vi "NM GlobalTest.vi"() -> ()   [LabVIEW 2010] (continued)
          n20 = Select(t=4, s="Timing", f=0) -> (s? t:f=w5836:i32)
        }
        frame 5 {
          # "TRIGGERING"
          n21 = Select(t=5, s="Trig", f=0) -> (s? t:f=w5841:i32)
        }
        frame 6 {
          # "START"
          n22 = Select(t=6, s="Start", f=0) -> (s? t:f=w5846:i32)
        }
        frame 7 {
          # "WRITE"
          n23 = Select(t=7, s="Write", f=0) -> (s? t:f=w5851:i32)
        }
        frame 8 {
          # "IDLE and UPDATE CONTROLS"
          n24 = Select(t=1, s="Idle 2", f=0) -> (s? t:f=w5856:i32)
        }
        frame 9 {
          # "READ"
          n25 = Select(t=11, s="Read", f=0) -> (s? t:f=w5861:i32)
        }
        frame 10 {
          # "START"
          n26 = Select(t=6, s="Start", f=0) -> (s? t:f=w5867:i32)
        }
        frame 11 {
          # "STATUS"
          n27 = Select(t=8, s="Status\nLoop", f=0) -> (s? t:f=w5873:i32)
        }
        frame 12 {
          # "Property Nodes"
          n28 = Select(t=13, s="Props", f=0) -> (s? t:f=w5877:i32)
        }
        frame 13 {
          # "WAIT"
          n29 = Select(t=12, s="Wait", f=0) -> (s? t:f=w5882:i32)
        }
        frame 14 {
          # "STOP"
          n30 = Select(t=9, s="Stop", f=0) -> (s? t:f=w5888:i32)
        }
        frame 15 {
          # "CLEAR"
          n31 = case shown="\"ULx\", Default" w5893 {
            tunnel: w5894 -> [w5900 _]
            tunnel: w5895 -> [_ w5903]
            frame "ULx", Default {
              n32 = call "ULxTaskInfo.vi"("task in"=w5900) -> ("Task"=w5901:i32)  [unwired: 2 out]
              n33 = local write "Task"(w5901) -> ()
            }
            frame "DAQmx" {
              n34 = call "DAQmxTaskInfo.vi"("task in"=w5903) -> ("Name"=w5902:refnum<k21>)  [unwired: 1 out]
              n35 = local write "Name"(w5902) -> ()
            }
          }
          n36 = call "TextError.vi"("error in"=w5891) -> ("message"=w5892:string)  [unwired: 1 in]
          n37 = local write "message 2"(w5892) -> ()
          n38 = Select(t=10, s="Clear", f=0) -> (s? t:f=w5897:i32)
        }
        frame 16 {
          # "Task Control"
          n39 = Select(t=14, s="NI\nTC", f=0) -> (s? t:f=w5904:i32)
        }
        frame 17 {
          n40 = case shown="True" "Clear\nError" {
            tunnel: w5910 -> [w5913 w5915]
            tunnel: [w5913 w5914] -> w5909
            frame False {
            }
            frame True {
              n41 = local write "Clear\nError"(FALSE) -> ()
              n42 = call <vilib>:"Clear Errors.vi"("error in (no error)"=w5915) -> ("error out"=w5914:errorcluster)  [unwired: 6 in]
            }
          }
        }
      }
      n43 = case shown="13" w33 {
        tunnel: "SelLib" -> [_ _ w155 w1018 w1069 w1147 w1386 w1435 w2708 w2768 w2791 w2812 w3897 w3943 w5784]
        tunnel: w22 -> [w47 w54 w153 w1024 w1068 w1148 w1395 w1434 w2714 w2767 w2794 w2815 w3901 w3940 w5788]
        tunnel: w23 -> [w46 w53 w154 w1023 w1067 w1150 w1394 w1433 w2713 w2766 w2793 w2814 w3902 w3941 w5786]
        tunnel: [w47 w52 w150 w1021 w1065 w1158 w1385 w1431 w2711 w2764 w2789 w2811 w3900 w3938 w5787] -> w35
        tunnel: [w46 w51 w151 w1020 w1064 w1157 w1384 w1430 w2710 w2763 w2788 w2810 w3899 w3937 w5783] -> w34
        tunnel: [w45 _ w152 w1019 w1063 w1156 w1383 w1429 w2709 w2762 w2787 w2809 w3898 w3939 w5782] -> w32
        tunnel: w16 -> [w45 _ _ w1022 w1066 w1149 w1393 w1432 w2712 w2765 w2792 w2813 w3903 w3942 w5785]
        tunnel: "Item" -> [_ _ w146 _ w1061 w1145 w1391 w1428 w2707 w2760 w2785 w2808 w3892 w3936 w5779]
        tunnel: w19 -> [_ w50 _ _ _ _ w1390 _ _ _ _ _ _ _ _]
        tunnel: w17 -> [w40 _ _ _ _ _ _ _ _ _ _ _ _ _ _]
        frame ..0, Default {
          # "Do Nothing"
          n44 = First Call?() -> (First Call?: T/F=w38:bool)
          n45 = Or(x=w38, y=w40) -> (x .or. y?=w39:bool)
          n46 = case shown="False" w39 {
            frame False {
            }
            frame True {
              n47 = local read "SelLib"() -> (w48:enum32{"ULx", "DAQmx"})
              n48 = local write "AChan"(w48) -> ()
              n49 = local write "TrgEdge"(w48) -> ()
              n50 = local write "DChan"(w48) -> ()
              n51 = local write "CtrChan"(w48) -> ()
              n52 = local write "CompIn"(w48) -> ()
              n53 = local write "CompOut"(w48) -> ()
              n54 = local write "TmgImp"(w48) -> ()
              n55 = local write "TmgWfm"(w48) -> ()
              n56 = local write "UDClock"(w48) -> ()
              n57 = local write "SetWProps"(w48) -> ()
              n58 = local write "GetWProps"(w48) -> ()
              n59 = local write "GetCOPrp"(w48) -> ()
              n60 = local write "TrigLib"(w48) -> ()
              n61 = local write "GetCiPrp"(w48) -> ()
              n62 = local write "GetTmgPrp"(w48) -> ()
            }
          }
          n63 = local read "Timing"() -> (w43:bool)
          n64 = local read "Write"() -> (w44:bool)
          n65 = local read "Props"() -> (w37:bool)
          n66 = local read "Trig"() -> (w42:bool)
          n67 = local read "Read"() -> (w41:bool)
          n68 = property on="GetSet" class="TabCtl (strict)"("Visible"=w37) -> ()  [unwired: 2 in, 2 out]
          n69 = property on="TrigType" class="TabCtl (strict)"("Visible"=w42) -> ()  [unwired: 2 in, 2 out]
          n70 = property on="Tab Control" class="TabCtl (strict)"("Visible"=w43) -> ()  [unwired: 2 in, 2 out]
          n71 = property on="TaskType 2" class="TabCtl (strict)"("Visible"=w44) -> ()  [unwired: 2 in, 2 out]
          n72 = property on="ReadType" class="TabCtl (strict)"("Visible"=w41) -> ()  [unwired: 2 in, 2 out]
        }
        frame 1 {
          # "IDLE and UPDATE CONTROLS"
          n73 = while {
            shift-right: [w80] -> _
            shift-left: _ -> [w97]
            tunnel: [FALSE ("f")] -> w49
            tunnel: w54 -> [w85]
            tunnel: w53 -> [w84]
            tunnel: [w79] -> w52
            tunnel: [w68] -> w51
            tunnel: w50 -> [w73]
            stop <- w100 stop-if-true
            n74 = case shown="0, Default" w73 {
              tunnel: ["Clear" "Clear"] -> w91
              tunnel: ["Stop" "Stop"] -> w90
              tunnel: ["Start" "Start"] -> w89
              frame 0, Default {
              }
              frame 1 {
              }
            }
            n75 = local read "SelLib"() -> (w69:enum32{"ULx", "DAQmx"})
            n76 = Not(x="Plots") -> (.not. x?=w58:bool)
            n77 = local write "UDClock"(w69) -> ()
            n78 = local write "TmgWfm"(w69) -> ()
            n79 = local write "TmgImp"(w69) -> ()
            n80 = property on="DblPlot" class="WFGraph (strict)"("Visible"="Plots") -> ()  [unwired: 2 in, 2 out]
            n81 = property on="u32Plot" class="WFGraph (strict)"("Visible"="Plots") -> ()  [unwired: 2 in, 2 out]
            n82 = property on="u32Array" class="Arr (strict)"("Visible"=w58) -> ()  [unwired: 2 in, 2 out]
            n83 = property on="DblArray 2" class="Arr (strict)"("Visible"=w58) -> ()  [unwired: 2 in, 2 out]
            n84 = call "NMIdleLoop.vi"("mx task in"=w85, "ULx task in"=w84, "Tab Control"=w69, "Start"=w89, "ExStop"=w90, "ExClear"=w91) -> ("Task Start"=w86:bool, "Task Stop"=w87:bool, "Task Clear"=w88:bool, "mx task out"=w79:refnum<k21>, "ULx task out"=w68:refnum<k24>, "Name"=w81:refnum<k21>, "Task"=w77:i32, "Function"=w82:i32, "error out"=w56:errorcluster)  [unwired: 5 in]
            n85 = Compound Arithmetic op=OR(w88, w87, w86) -> (w83:bool)
            n86 = local write "TrgEdge"(w69) -> ()
            n87 = local write "AChan"(w69) -> ()
            n88 = local write "CompOut"(w69) -> ()
            n89 = local write "Name"(w81) -> ()
            n90 = local read "Write"() -> (w92:bool)
            n91 = local read "Read"() -> (w74:bool)
            n92 = local read "Timing"() -> (w76:bool)
            n93 = local read "Trig"() -> (w75:bool)
            n94 = local write "CtrChan"(w69) -> ()
            n95 = local write "DChan"(w69) -> ()
            n96 = local write "CompIn"(w69) -> ()
            n97 = property on="ReadType" class="TabCtl (strict)"("Visible"=w74) -> ()  [unwired: 2 in, 2 out]
            n98 = property on="TaskType 2" class="TabCtl (strict)"("Visible"=w92) -> ()  [unwired: 2 in, 2 out]
            n99 = property on="Tab Control" class="TabCtl (strict)"("Visible"=w76) -> ()  [unwired: 2 in, 2 out]
            n100 = property on="TrigType" class="TabCtl (strict)"("Visible"=w75) -> ()  [unwired: 2 in, 2 out]
            n101 = local write "Task"(w77) -> ()
            n102 = case shown="\"DAQmx\"" w69 {
              tunnel: w79 -> [_ w125]
              tunnel: w77 -> [w117 _]
              tunnel: w68 -> [w116 _]
              tunnel: [w112 w120] -> w57
              tunnel: w56 -> [w111 w123]
              tunnel: [w110 w124] -> w55
              frame "ULx", Default {
                n103 = Equal To 0?(x=w117) -> (x = 0?=w118:bool)
                n104 = call <vilib>:"ULx Is Task Done.vi"("task in"=w116, "error in"=w111) -> ("task done?"=w115:bool, "error out"=w110:errorcluster)  [unwired: 11 in, 1 out]
                n105 = local write "Task Cleared"(w118) -> ()
                n106 = local write "Task Stopped"(w115) -> ()
                n107 = Unbundle By Name(w110) -> ("code"=w114:i32)
                n108 = Not Equal?(x=w114, y=100000) -> (x != y?=w112:bool)
              }
              frame "DAQmx" {
                n109 = call <vilib>:"DAQmx Is Task Done.vi"("task/channels in"=w125, "error in"=w123) -> ("task done?"=w122:bool, "error out"=w124:errorcluster)  [unwired: 11 in, 1 out]
                n110 = Unbundle By Name(w124) -> ("code"=w127:i32)
                n111 = Equal?(x=w127, y=-200088) -> (x = y?=w119:bool)
                n112 = Or(x=w122, y=w119) -> (x .or. y?=w121:bool)
                n113 = Not(x=w119) -> (.not. x?=w120:bool)
                n114 = local write "Task Stopped"(w121) -> ()
                n115 = local write "Task Cleared"(w119) -> ()
              }
            }
            n116 = case shown="0, Default" w82 {
              tunnel: w69 -> [_ w129 w132 _]
              tunnel: w77 -> [_ _ _ _]
              frame 0, Default {
              }
              frame 1 {
                w128 = FALSE ("Start 2")
                n117 = case shown="\"ULx\", Default" w129 {
                  frame "ULx", Default {
                    n118 = local write "Task Stopped"(FALSE ("Task Stopped")) -> ()
                  }
                  frame "DAQmx" {
                  }
                }
                n119 = local write "Start"(w128) -> ()
                n120 = local write "Start"(w128) -> ()
              }
              frame 2 {
                w131 = FALSE ("Stop")
                n121 = case shown="\"ULx\", Default" w132 {
                  frame "ULx", Default {
                    n122 = local write "Task Stopped"(TRUE ("Task Stopped")) -> ()
                  }
                  frame "DAQmx" {
                  }
                }
                n123 = local write "Stop"(w131) -> ()
                n124 = local write "Stop"(w131) -> ()
              }
              frame 3 {
                w134 = FALSE ("Clear")
                n125 = local write "Clear"(w134) -> ()
                n126 = local write "Clear"(w134) -> ()
              }
            }
            n127 = local write "GetWProps"(w69) -> ()
            n128 = local write "SetWProps"(w69) -> ()
            n129 = local write "TrigLib"(w69) -> ()
            n130 = local read "Mod Array"() -> (w64:bool)
            n131 = local write "GetTmgPrp"(w69) -> ()
            n132 = local write "GetCOPrp"(w69) -> ()
            n133 = property on="digital data 3" class="Arr (strict)"("Visible"="Dig/Ctr") -> ()  [unwired: 2 in, 2 out]
            n134 = local write "GetCiPrp"(w69) -> ()
            n135 = property on="DataGen" class="TabCtl (strict)"("Visible"="Data") -> ()  [unwired: 2 in, 2 out]
            n136 = property on="Tab Control 3" class="TabCtl (strict)"("Visible"=w64) -> ()  [unwired: 2 in, 2 out]
            n137 = Not(x="Dig/Ctr") -> (.not. x?=w61:bool)
            n138 = local read "Idle 2"() -> (w71:bool)
            n139 = local read "Idle"() -> (w78:bool)
            n140 = local read "Props"() -> (w70:bool)
            n141 = Not(x=w97) -> (.not. x?=w95:bool)
            n142 = property on="counter data" class="Arr (strict)"("Visible"=w61) -> ()  [unwired: 2 in, 2 out]
            n143 = Wait Until Next ms Multiple(millisecond multiple=u32 200) -> ()  [unwired: 1 out]
            n144 = property on="GetSet" class="TabCtl (strict)"("Visible"=w70) -> ()  [unwired: 2 in, 2 out]
            n145 = Or(x=w71, y=w78) -> (x .or. y?=w72:bool)
            n146 = case shown="Error" w55 {
              selector: w55 -> [w135 w140]
              tunnel: w83 -> [w136 _]
              tunnel: w57 -> [_ w139]
              frame No Error {
                n147 = case shown="True" w136 {
                  tunnel: w135 -> [_ w138]
                  frame False {
                  }
                  frame True {
                    n148 = call "TextError.vi"("error in"=w138) -> ("message"=w137:string)  [unwired: 1 in]
                    n149 = local write "message 2"(w137) -> ()
                  }
                }
              }
              frame Error {
                n150 = case shown="True" w139 {
                  tunnel: w140 -> [_ w142]
                  frame False {
                  }
                  frame True {
                    n151 = call "TextError.vi"("error in"=w142) -> ("message"=w141:string)  [unwired: 1 in]
                    n152 = local write "message 2"(w141) -> ()
                  }
                }
              }
            }
            n153 = local read "stop"() -> (w96:bool)
            n154 = Not(x=w72) -> (.not. x?=w98:bool)
            n155 = Select(t=w95, s=w72, f=FALSE) -> (s? t:f=w80:bool)
            n156 = Not(x="Show Plot") -> (.not. x?=w62:bool)
            n157 = Not(x="Show Plot") -> (.not. x?=w65:bool)
            n158 = property on="DblArray" class="WFGraph (strict)"("Visible"="Show Plot") -> ()  [unwired: 2 in, 2 out]
            n159 = case shown="0, Default" w73 {
              tunnel: w80 -> [w108 w109]
              frame 0, Default {
                "Idle" <- w108
              }
              frame 1 {
                "Idle 3" <- w109
              }
            }
            n160 = property on="data 41" class="Arr (strict)"("Visible"=w65) -> ()  [unwired: 2 in, 2 out]
            n161 = Compound Arithmetic op=OR(w96, w98, "Submit") -> (w100:bool)
            n162 = property on="data 7" class="Arr (strict)"("Visible"=w62) -> ()  [unwired: 2 in, 2 out]
            n163 = property on="data 76" class="WFGraph (strict)"("Visible"="Show Plot") -> ()  [unwired: 2 in, 2 out]
          }
          n164 = local write "Idle"(w49) -> ()
          n165 = local write "Idle 3"(w49) -> ()
          n166 = local write "Submit"(w49) -> ()
        }
        frame 2 {
          # "CREATE CHANNELS"
          n167 = case shown="\"Counter\"" "TaskType" {
            tunnel: [w169 w401 w483 w835 w948] -> w151
            tunnel: [w168 w400 w485 w836 w950] -> w149
            tunnel: [w167 w399 w484 w837 w949] -> w148
            tunnel: w155 -> [w166 w398 w482 _ _]
            tunnel: [w165 w397 w481 w834 w947] -> w150
            tunnel: w153 -> [w164 w395 w480 w834 w947]
            tunnel: w154 -> [w163 w396 w479 _ _]
            tunnel: [w162 w394 w478 w833 w946] -> w143
            frame "Analog", Default {
              n168 = case shown="\"DAQmx\"" w166 {
                tunnel: [w176 w279] -> w169
                tunnel: [w175 w282] -> w168
                tunnel: [w174 w281] -> w167
                tunnel: [w173 w280] -> w165
                tunnel: w164 -> [w173 _]
                tunnel: w163 -> [_ w279]
                tunnel: [w172 ""] -> w162
                tunnel: [w171 w277] -> w157
                tunnel: [w170 w276] -> w156
                frame "ULx", Default {
                  n169 = case shown="\"AO Volts\"" "AnalogType" {
                    tunnel: [w183 w210 w228 w247 w266] -> w174
                    tunnel: [w182 w211 w229 w248 w267] -> w175
                    tunnel: [w181 w217 w235 w254 w273] -> w176
                    tunnel: ["ULx" "ULx" "ULx" "ULx" "ULx"] -> w172
                    tunnel: [-5.0 ("min") -5.0 ("min") -5.0 ("min") "min" "min"] -> w170
                    tunnel: [5.0 ("max") 5.0 ("max") 5.0 ("max") "max" "max"] -> w171
                    frame "AI Volts", Default {
                      n170 = call-poly <vilib>:"ULx Create Virtual Channel.vi"("maximum value"="max", "minimum value"="min", "physical channels"="ULx") -> ("task out"=w198:refnum<k24>, "error out"=w188:errorcluster)  [unwired: 11 in]
                      n171 = call "TrapBlankChan.vi"("error in (no error)"=w188) -> ("error out"=w187:errorcluster)  [unwired: 9 in, 1 out]
                      n172 = call-poly <vilib>:"ULx Create Virtual Channel.vi"("task in"=w198, "maximum value"="max 2", "minimum value"="min 2", "physical channels"="physical channels 2", "error in"=w187) -> ("task out"=w197:refnum<k24>, "error out"=w186:errorcluster)  [unwired: 9 in]
                      n173 = call "TrapBlankChan.vi"("error in (no error)"=w186) -> ("error out"=w185:errorcluster)  [unwired: 9 in, 1 out]
                      n174 = call-poly <vilib>:"ULx Create Virtual Channel.vi"("task in"=w197, "maximum value"="max 3", "minimum value"="min 3", "physical channels"="physical channels 3", "error in"=w185) -> ("task out"=w181:refnum<k24>, "error out"=w184:errorcluster)  [unwired: 9 in]
                      n175 = call "TrapBlankChan.vi"("error in (no error)"=w184) -> ("message"=w183:string, "error out"=w182:errorcluster)  [unwired: 9 in]
                    }
                    frame "AI Cur" {
                      n176 = call-poly <vilib>:"ULx Create Virtual Channel.vi"("maximum value"="max", "minimum value"="min", "physical channels"="ULx") -> ("task out"=w219:refnum<k24>, "error out"=w216:errorcluster)  [unwired: 11 in]
                      n177 = call "TrapBlankChan.vi"("error in (no error)"=w216) -> ("error out"=w215:errorcluster)  [unwired: 9 in, 1 out]
                      n178 = call-poly <vilib>:"ULx Create Virtual Channel.vi"("task in"=w219, "maximum value"="max 4", "minimum value"="min 4", "physical channels"="physical channels 5", "error in"=w215) -> ("task out"=w218:refnum<k24>, "error out"=w214:errorcluster)  [unwired: 9 in]
                      n179 = call "TrapBlankChan.vi"("error in (no error)"=w214) -> ("error out"=w213:errorcluster)  [unwired: 9 in, 1 out]
                      n180 = call-poly <vilib>:"ULx Create Virtual Channel.vi"("task in"=w218, "maximum value"="max 5", "minimum value"="min 5", "physical channels"="physical channels 6", "error in"=w213) -> ("task out"=w217:refnum<k24>, "error out"=w212:errorcluster)  [unwired: 9 in]
                      n181 = call "TrapBlankChan.vi"("error in (no error)"=w212) -> ("message"=w210:string, "error out"=w211:errorcluster)  [unwired: 9 in]
                    }
                    frame "AI Temp" {
                      n182 = call-poly <vilib>:"ULx Create Virtual Channel.vi"("physical channels"="ULx", "units"="units") -> ("task out"=w237:refnum<k24>, "error out"=w234:errorcluster)  [unwired: 12 in]
                      n183 = call "TrapBlankChan.vi"("error in (no error)"=w234) -> ("error out"=w233:errorcluster)  [unwired: 9 in, 1 out]
                      n184 = call-poly <vilib>:"ULx Create Virtual Channel.vi"("task in"=w237, "physical channels"="physical channels 8", "units"="units 2", "error in"=w233) -> ("task out"=w236:refnum<k24>, "error out"=w232:errorcluster)  [unwired: 10 in]
                      n185 = call "TrapBlankChan.vi"("error in (no error)"=w232) -> ("error out"=w231:errorcluster)  [unwired: 9 in, 1 out]
                      n186 = call-poly <vilib>:"ULx Create Virtual Channel.vi"("task in"=w236, "physical channels"="physical channels 9", "units"="units 3", "error in"=w231) -> ("task out"=w235:refnum<k24>, "error out"=w230:errorcluster)  [unwired: 10 in]
                      n187 = call "TrapBlankChan.vi"("error in (no error)"=w230) -> ("message"=w228:string, "error out"=w229:errorcluster)  [unwired: 9 in]
                    }
                    frame "AO Volts" {
                      n188 = call-poly <vilib>:"ULx Create Virtual Channel.vi"("maximum value"="max", "minimum value"="min", "physical channels"="ULx") -> ("task out"=w256:refnum<k24>, "error out"=w253:errorcluster)  [unwired: 11 in]
                      n189 = call "TrapBlankChan.vi"("error in (no error)"=w253) -> ("error out"=w252:errorcluster)  [unwired: 9 in, 1 out]
                      n190 = call-poly <vilib>:"ULx Create Virtual Channel.vi"("task in"=w256, "maximum value"="max 8", "minimum value"="min 8", "physical channels"="physical channels 11", "error in"=w252) -> ("task out"=w255:refnum<k24>, "error out"=w251:errorcluster)  [unwired: 9 in]
                      n191 = call "TrapBlankChan.vi"("error in (no error)"=w251) -> ("error out"=w250:errorcluster)  [unwired: 9 in, 1 out]
                      n192 = call-poly <vilib>:"ULx Create Virtual Channel.vi"("task in"=w255, "maximum value"="max 7", "minimum value"="min 7", "physical channels"="physical channels 12", "error in"=w250) -> ("task out"=w254:refnum<k24>, "error out"=w249:errorcluster)  [unwired: 9 in]
                      n193 = call "TrapBlankChan.vi"("error in (no error)"=w249) -> ("message"=w247:string, "error out"=w248:errorcluster)  [unwired: 9 in]
                    }
                    frame "AO Cur" {
                      n194 = call-poly <vilib>:"ULx Create Virtual Channel.vi"("maximum value"="max", "minimum value"="min", "physical channels"="ULx") -> ("task out"=w275:refnum<k24>, "error out"=w272:errorcluster)  [unwired: 11 in]
                      n195 = call "TrapBlankChan.vi"("error in (no error)"=w272) -> ("error out"=w271:errorcluster)  [unwired: 9 in, 1 out]
                      n196 = call-poly <vilib>:"ULx Create Virtual Channel.vi"("task in"=w275, "maximum value"="max 11", "minimum value"="min 11", "physical channels"="physical channels 14", "error in"=w271) -> ("task out"=w274:refnum<k24>, "error out"=w270:errorcluster)  [unwired: 9 in]
                      n197 = call "TrapBlankChan.vi"("error in (no error)"=w270) -> ("error out"=w269:errorcluster)  [unwired: 9 in, 1 out]
                      n198 = call-poly <vilib>:"ULx Create Virtual Channel.vi"("task in"=w274, "maximum value"="max 10", "minimum value"="min 10", "physical channels"="physical channels 15", "error in"=w269) -> ("task out"=w273:refnum<k24>, "error out"=w268:errorcluster)  [unwired: 9 in]
                      n199 = call "TrapBlankChan.vi"("error in (no error)"=w268) -> ("message"=w266:string, "error out"=w267:errorcluster)  [unwired: 9 in]
                    }
                  }
                }
                frame "DAQmx" {
                  n200 = case shown="\"AI Volts\", Default" "xAnalog\nType" {
                    tunnel: [w289 w316 w344 w373 w392] -> w281
                    tunnel: [w290 w317 w350 w374 w393] -> w282
                    tunnel: [w292 w324 w349 w367 w388] -> w280
                    tunnel: [5.0 ("max") 5.0 ("max") 5.0 ("max") "max" "max"] -> w277
                    tunnel: [-5.0 ("min") -5.0 ("min") -5.0 ("min") "min" "min"] -> w276
                    frame "AI Volts", Default {
                      n201 = call-poly <vilib>:"DAQmx Create Virtual Channel.vi"("maximum value"="max", "minimum value"="min", "physical channels"="DAQmx", "name to assign"="name 1") -> ("task out"=w302:refnum<k21>, "error out"=w307:errorcluster)  [unwired: 10 in]
                      n202 = call "NITrapBlankChan.vi"("error in (no error)"=w307) -> ("error out"=w303:errorcluster)  [unwired: 9 in, 1 out]
                      n203 = call-poly <vilib>:"DAQmx Create Virtual Channel.vi"("task in"=w302, "maximum value"="max 19", "minimum value"="min 19", "physical channels"="physical channels 32", "name to assign"="name 2", "error in"=w303) -> ("task out"=w298:refnum<k21>, "error out"=w297:errorcluster)  [unwired: 8 in]
                      n204 = call "NITrapBlankChan.vi"("error in (no error)"=w297) -> ("error out"=w296:errorcluster)  [unwired: 9 in, 1 out]
                      n205 = call-poly <vilib>:"DAQmx Create Virtual Channel.vi"("task in"=w298, "maximum value"="max 20", "minimum value"="min 20", "physical channels"="physical channels 33", "name to assign"="name 3", "error in"=w296) -> ("task out"=w292:refnum<k21>, "error out"=w291:errorcluster)  [unwired: 8 in]
                      n206 = call "NITrapBlankChan.vi"("error in (no error)"=w291) -> ("message"=w289:string, "error out"=w290:errorcluster)  [unwired: 9 in]
                    }
                    frame "AI Cur" {
                      n207 = call-poly <vilib>:"DAQmx Create Virtual Channel.vi"("maximum value"="max", "minimum value"="min", "physical channels"="DAQmx") -> ("task out"=w325:refnum<k21>, "error out"=w322:errorcluster)  [unwired: 11 in]
                      n208 = call "NITrapBlankChan.vi"("error in (no error)"=w322) -> ("error out"=w321:errorcluster)  [unwired: 9 in, 1 out]
                      n209 = call-poly <vilib>:"DAQmx Create Virtual Channel.vi"("task in"=w325, "maximum value"="max 22", "minimum value"="min 22", "physical channels"="physical channels 35", "error in"=w321) -> ("task out"=w323:refnum<k21>, "error out"=w320:errorcluster)  [unwired: 9 in]
                      n210 = call "NITrapBlankChan.vi"("error in (no error)"=w320) -> ("error out"=w319:errorcluster)  [unwired: 9 in, 1 out]
                      n211 = call-poly <vilib>:"DAQmx Create Virtual Channel.vi"("task in"=w323, "maximum value"="max 23", "minimum value"="min 23", "physical channels"="physical channels 36", "error in"=w319) -> ("task out"=w324:refnum<k21>, "error out"=w318:errorcluster)  [unwired: 9 in]
                      n212 = call "NITrapBlankChan.vi"("error in (no error)"=w318) -> ("message"=w316:string, "error out"=w317:errorcluster)  [unwired: 9 in]
                    }
                    frame "AI Temp" {
                      n213 = call-poly <vilib>:"DAQmx Create Virtual Channel.vi"("maximum value"="max", "minimum value"="min", "physical channels"="DAQmx", "name to assign"="Names", "units"="units") -> ("task out"=w348:refnum<k21>, "error out"=w355:errorcluster)  [unwired: 9 in]
                      n214 = call "NITrapBlankChan.vi"("error in (no error)"=w355) -> ("error out"=w354:errorcluster)  [unwired: 9 in, 1 out]
                      n215 = call-poly <vilib>:"DAQmx Create Virtual Channel.vi"("task in"=w348, "maximum value"="max 25", "minimum value"="min 25", "physical channels"="physical channels 38", "name to assign"="T2", "units"="units 13", "error in"=w354) -> ("task out"=w347:refnum<k21>, "error out"=w353:errorcluster)  [unwired: 7 in]
                      n216 = call "NITrapBlankChan.vi"("error in (no error)"=w353) -> ("error out"=w352:errorcluster)  [unwired: 9 in, 1 out]
                      n217 = call-poly <vilib>:"DAQmx Create Virtual Channel.vi"("task in"=w347, "maximum value"="max 26", "minimum value"="min 26", "physical channels"="physical channels 39", "name to assign"="T3", "units"="units 15", "error in"=w352) -> ("task out"=w349:refnum<k21>, "error out"=w351:errorcluster)  [unwired: 7 in]
                      n218 = call "NITrapBlankChan.vi"("error in (no error)"=w351) -> ("message"=w344:string, "error out"=w350:errorcluster)  [unwired: 9 in]
                    }
                    frame "AO Volts" {
                      n219 = call-poly <vilib>:"DAQmx Create Virtual Channel.vi"("maximum value"="max", "minimum value"="min", "physical channels"="DAQmx") -> ("task out"=w369:refnum<k21>, "error out"=w372:errorcluster)  [unwired: 11 in]
                      n220 = call "NITrapBlankChan.vi"("error in (no error)"=w372) -> ("error out"=w370:errorcluster)  [unwired: 9 in, 1 out]
                      n221 = call-poly <vilib>:"DAQmx Create Virtual Channel.vi"("task in"=w369, "maximum value"="max 28", "minimum value"="min 28", "physical channels"="physical channels 41", "error in"=w370) -> ("task out"=w365:refnum<k21>, "error out"=w364:errorcluster)  [unwired: 9 in]
                      n222 = call "NITrapBlankChan.vi"("error in (no error)"=w364) -> ("error out"=w368:errorcluster)  [unwired: 9 in, 1 out]
                      n223 = call-poly <vilib>:"DAQmx Create Virtual Channel.vi"("task in"=w365, "maximum value"="max 29", "minimum value"="min 29", "physical channels"="physical channels 42", "error in"=w368) -> ("task out"=w367:refnum<k21>, "error out"=w366:errorcluster)  [unwired: 9 in]
                      n224 = call "NITrapBlankChan.vi"("error in (no error)"=w366) -> ("message"=w373:string, "error out"=w374:errorcluster)  [unwired: 9 in]
                    }
                    frame "AO Cur" {
                      n225 = call-poly <vilib>:"DAQmx Create Virtual Channel.vi"("maximum value"="max", "minimum value"="min", "physical channels"="DAQmx") -> ("task out"=w389:refnum<k21>, "error out"=w391:errorcluster)  [unwired: 11 in]
                      n226 = call "NITrapBlankChan.vi"("error in (no error)"=w391) -> ("error out"=w386:errorcluster)  [unwired: 9 in, 1 out]
                      n227 = call-poly <vilib>:"DAQmx Create Virtual Channel.vi"("task in"=w389, "maximum value"="max 31", "minimum value"="min 31", "physical channels"="physical channels 44", "error in"=w386) -> ("task out"=w387:refnum<k21>, "error out"=w385:errorcluster)  [unwired: 9 in]
                      n228 = call "NITrapBlankChan.vi"("error in (no error)"=w385) -> ("error out"=w384:errorcluster)  [unwired: 9 in, 1 out]
                      n229 = call-poly <vilib>:"DAQmx Create Virtual Channel.vi"("task in"=w387, "maximum value"="max 32", "minimum value"="min 32", "physical channels"="physical channels 45", "error in"=w384) -> ("task out"=w388:refnum<k21>, "error out"=w383:errorcluster)  [unwired: 9 in]
                      n230 = call "NITrapBlankChan.vi"("error in (no error)"=w383) -> ("message"=w392:string, "error out"=w393:errorcluster)  [unwired: 9 in]
                    }
                  }
                }
              }
              n231 = Multiply(x=w157, y=1.01) -> (x*y=w159:dbl)
              n232 = Multiply(x=1.01, y=w156) -> (x*y=w158:dbl)
              n233 = property on="data 2" class="Slide (strict)"("Scale.Maximum"=w159) -> ()  [unwired: 2 in, 2 out]
              n234 = property on="data 2" class="Slide (strict)"("Scale.Minimum"=w158) -> ()  [unwired: 2 in, 2 out]
            }
            frame "Digital" {
              n235 = case shown="\"ULx\", Default" w398 {
                tunnel: [w406 w442] -> w401
                tunnel: [w405 w445] -> w400
                tunnel: [w404 w444] -> w399
                tunnel: [w403 w443] -> w397
                tunnel: w396 -> [_ w442]
                tunnel: w395 -> [w403 _]
                tunnel: [w402 ""] -> w394
                frame "ULx", Default {
                  n236 = case shown="\"Digital Input\", Default" "DigitalType" {
                    tunnel: [w416 w430] -> w404
                    tunnel: [w415 w431] -> w405
                    tunnel: [w414 w437] -> w406
                    tunnel: ["ULx" "ULx"] -> w402
                    frame "Digital Input", Default {
                      n237 = call-poly <vilib>:"ULx Create Virtual Channel.vi"("lines"="ULx", "line grouping"="line grouping") -> ("task out"=w423:refnum<k24>, "error out"=w421:errorcluster)  [unwired: 12 in]
                      n238 = call "TrapBlankChan.vi"("error in (no error)"=w421) -> ("error out"=w420:errorcluster)  [unwired: 9 in, 1 out]
                      n239 = call-poly <vilib>:"ULx Create Virtual Channel.vi"("task in"=w423, "lines"="lines 2", "line grouping"="line grouping 2", "error in"=w420) -> ("task out"=w422:refnum<k24>, "error out"=w419:errorcluster)  [unwired: 10 in]
                      n240 = call "TrapBlankChan.vi"("error in (no error)"=w419) -> ("error out"=w418:errorcluster)  [unwired: 9 in, 1 out]
                      n241 = call-poly <vilib>:"ULx Create Virtual Channel.vi"("task in"=w422, "lines"="lines 3", "line grouping"="line grouping 3", "error in"=w418) -> ("task out"=w414:refnum<k24>, "error out"=w417:errorcluster)  [unwired: 10 in]
                      n242 = call "TrapBlankChan.vi"("error in (no error)"=w417) -> ("message"=w416:string, "error out"=w415:errorcluster)  [unwired: 9 in]
                    }
                    frame "Digital Output" {
                      n243 = call-poly <vilib>:"ULx Create Virtual Channel.vi"("lines"="ULx", "line grouping"="line grouping") -> ("task out"=w439:refnum<k24>, "error out"=w436:errorcluster)  [unwired: 12 in]
                      n244 = call "TrapBlankChan.vi"("error in (no error)"=w436) -> ("error out"=w435:errorcluster)  [unwired: 9 in, 1 out]
                      n245 = call-poly <vilib>:"ULx Create Virtual Channel.vi"("task in"=w439, "lines"="lines 5", "line grouping"="line grouping 5", "error in"=w435) -> ("task out"=w438:refnum<k24>, "error out"=w434:errorcluster)  [unwired: 10 in]
                      n246 = call "TrapBlankChan.vi"("error in (no error)"=w434) -> ("error out"=w433:errorcluster)  [unwired: 9 in, 1 out]
                      n247 = call-poly <vilib>:"ULx Create Virtual Channel.vi"("task in"=w438, "lines"="lines 6", "line grouping"="line grouping 6", "error in"=w433) -> ("task out"=w437:refnum<k24>, "error out"=w432:errorcluster)  [unwired: 10 in]
                      n248 = call "TrapBlankChan.vi"("error in (no error)"=w432) -> ("message"=w430:string, "error out"=w431:errorcluster)  [unwired: 9 in]
                    }
                  }
                }
                frame "DAQmx" {
                  n249 = case shown="..\"Digital Input\"" "xDigitalType" {
                    tunnel: [w446 w462] -> w444
                    tunnel: [w447 w469] -> w445
                    tunnel: [w448 w476] -> w443
                    frame .."Digital Input" {
                      n250 = call-poly <vilib>:"DAQmx Create Virtual Channel.vi"("lines"="DAQmx", "line grouping"="line grouping 4") -> ("task out"=w459:refnum<k21>, "error out"=w461:errorcluster)  [unwired: 12 in]
                      n251 = call "NITrapBlankChan.vi"("error in (no error)"=w461) -> ("error out"=w460:errorcluster)  [unwired: 9 in, 1 out]
                      n252 = call-poly <vilib>:"DAQmx Create Virtual Channel.vi"("task in"=w459, "lines"="lines 8", "line grouping"="line grouping 7", "error in"=w460) -> ("task out"=w458:refnum<k21>, "error out"=w457:errorcluster)  [unwired: 10 in]
                      n253 = call "NITrapBlankChan.vi"("error in (no error)"=w457) -> ("error out"=w456:errorcluster)  [unwired: 9 in, 1 out]
                      n254 = call-poly <vilib>:"DAQmx Create Virtual Channel.vi"("task in"=w458, "lines"="lines 9", "line grouping"="line grouping 8", "error in"=w456) -> ("task out"=w448:refnum<k21>, "error out"=w455:errorcluster)  [unwired: 10 in]
                      n255 = call "NITrapBlankChan.vi"("error in (no error)"=w455) -> ("message"=w446:string, "error out"=w447:errorcluster)  [unwired: 9 in]
                    }
                    frame "Digital Output".. {
                      n256 = call-poly <vilib>:"DAQmx Create Virtual Channel.vi"("lines"="DAQmx", "line grouping"="line grouping 9") -> ("task out"=w477:refnum<k21>, "error out"=w474:errorcluster)  [unwired: 12 in]
                      n257 = call "NITrapBlankChan.vi"("error in (no error)"=w474) -> ("error out"=w473:errorcluster)  [unwired: 9 in, 1 out]
                      n258 = call-poly <vilib>:"DAQmx Create Virtual Channel.vi"("task in"=w477, "lines"="lines 11", "line grouping"="line grouping 10", "error in"=w473) -> ("task out"=w475:refnum<k21>, "error out"=w472:errorcluster)  [unwired: 10 in]
                      n259 = call "NITrapBlankChan.vi"("error in (no error)"=w472) -> ("error out"=w471:errorcluster)  [unwired: 9 in, 1 out]
                      n260 = call-poly <vilib>:"DAQmx Create Virtual Channel.vi"("task in"=w475, "lines"="lines 12", "line grouping"="line grouping 11", "error in"=w471) -> ("task out"=w476:refnum<k21>, "error out"=w470:errorcluster)  [unwired: 10 in]
                      n261 = call "NITrapBlankChan.vi"("error in (no error)"=w470) -> ("message"=w462:string, "error out"=w469:errorcluster)  [unwired: 9 in]
                    }
                  }
                }
              }
            }
            frame "Counter" {
              n262 = case shown="\"ULx\", Default" w482 {
                tunnel: [w490 w627] -> w485
                tunnel: [w489 w628] -> w484
                tunnel: [w488 w625] -> w483
                tunnel: [w487 w626] -> w481
                tunnel: w480 -> [w487 _]
                tunnel: w479 -> [_ w625]
                tunnel: [w486 ""] -> w478
                frame "ULx", Default {
                  n263 = case shown="\"Freq Out\"" "CounterType" {
                    tunnel: [w506 w526 w548 w562 w576 w595 w614] -> w489
                    tunnel: [w505 w527 w549 w563 w577 w596 w615] -> w490
                    tunnel: [w504 w533 w555 w566 w583 w597 w616] -> w488
                    tunnel: ["ULx" "ULx" "ULx" "ULx" "ULx" "ULx" "ULx"] -> w486
                    frame "Freq In", Default {
                      n264 = call-poly <vilib>:"ULx Create Virtual Channel.vi"("counters"="ULx", "units"="units", "starting edge"="starting edge", "measurement time"="measure time") -> ("task out"=w513:refnum<k24>, "error out"=w511:errorcluster)  [unwired: 10 in]
                      n265 = call "TrapBlankChan.vi"("error in (no error)"=w511) -> ("error out"=w510:errorcluster)  [unwired: 9 in, 1 out]
                      n266 = call-poly <vilib>:"ULx Create Virtual Channel.vi"("task in"=w513, "counters"="counters 2", "units"="units 5", "error in"=w510, "starting edge"="starting edge 2", "measurement time"="measure time 2") -> ("task out"=w512:refnum<k24>, "error out"=w509:errorcluster)  [unwired: 8 in]
                      n267 = call "TrapBlankChan.vi"("error in (no error)"=w509) -> ("error out"=w508:errorcluster)  [unwired: 9 in, 1 out]
                      n268 = call-poly <vilib>:"ULx Create Virtual Channel.vi"("task in"=w512, "counters"="counters 3", "units"="units 6", "error in"=w508, "starting edge"="starting edge 3", "measurement time"="measure time 3") -> ("task out"=w504:refnum<k24>, "error out"=w507:errorcluster)  [unwired: 8 in]
                      n269 = call "TrapBlankChan.vi"("error in (no error)"=w507) -> ("message"=w506:string, "error out"=w505:errorcluster)  [unwired: 9 in]
                    }
                    frame "Period In" {
                      n270 = call-poly <vilib>:"ULx Create Virtual Channel.vi"("counters"="ULx", "units"="units", "starting edge"="starting edge", "measurement time"="measure time") -> ("task out"=w535:refnum<k24>, "error out"=w532:errorcluster)  [unwired: 10 in]
                      n271 = call "TrapBlankChan.vi"("error in (no error)"=w532) -> ("error out"=w531:errorcluster)  [unwired: 9 in, 1 out]
                      n272 = call-poly <vilib>:"ULx Create Virtual Channel.vi"("task in"=w535, "counters"="counters 5", "units"="units 8", "error in"=w531, "starting edge"="starting edge 5", "measurement time"="measure time 4") -> ("task out"=w534:refnum<k24>, "error out"=w530:errorcluster)  [unwired: 8 in]
                      n273 = call "TrapBlankChan.vi"("error in (no error)"=w530) -> ("error out"=w529:errorcluster)  [unwired: 9 in, 1 out]
                      n274 = call-poly <vilib>:"ULx Create Virtual Channel.vi"("task in"=w534, "counters"="counters 6", "units"="units 9", "error in"=w529, "starting edge"="starting edge 6", "measurement time"="measure time 5") -> ("task out"=w533:refnum<k24>, "error out"=w528:errorcluster)  [unwired: 8 in]
                      n275 = call "TrapBlankChan.vi"("error in (no error)"=w528) -> ("message"=w526:string, "error out"=w527:errorcluster)  [unwired: 9 in]
                    }
                    frame "Edge In" {
                      n276 = call-poly <vilib>:"ULx Create Virtual Channel.vi"("initial count"="initial count", "count direction"="direction", "edge"="edge", "counters"="ULx") -> ("task out"=w557:refnum<k24>, "error out"=w554:errorcluster)  [unwired: 10 in]
                      n277 = call "TrapBlankChan.vi"("error in (no error)"=w554) -> ("error out"=w553:errorcluster)  [unwired: 9 in, 1 out]
                      n278 = call-poly <vilib>:"ULx Create Virtual Channel.vi"("task in"=w557, "initial count"="initial count 2", "count direction"="direction 2", "edge"="edge 2", "counters"="counters 8", "error in"=w553) -> ("task out"=w556:refnum<k24>, "error out"=w552:errorcluster)  [unwired: 8 in]
                      n279 = call "TrapBlankChan.vi"("error in (no error)"=w552) -> ("error out"=w551:errorcluster)  [unwired: 9 in, 1 out]
                      n280 = call-poly <vilib>:"ULx Create Virtual Channel.vi"("task in"=w556, "initial count"="initial count 3", "count direction"="direction 3", "edge"="edge 3", "counters"="counters 9", "error in"=w551) -> ("task out"=w555:refnum<k24>, "error out"=w550:errorcluster)  [unwired: 8 in]
                      n281 = call "TrapBlankChan.vi"("error in (no error)"=w550) -> ("message"=w548:string, "error out"=w549:errorcluster)  [unwired: 9 in]
                    }
                    frame "Position In" {
                      n282 = call-poly <vilib>:"ULx Create Virtual Channel.vi"("counters"="ULx") -> ("task out"=w560:refnum<k24>, "error out"=w565:errorcluster)  [unwired: 13 in]
                      n283 = call "TrapBlankChan.vi"("error in (no error)"=w565) -> ("error out"=w561:errorcluster)  [unwired: 9 in, 1 out]
                      n284 = call-poly <vilib>:"ULx Create Virtual Channel.vi"("task in"=w560, "counters"="counters 11", "error in"=w561) -> ("task out"=w566:refnum<k24>, "error out"=w564:errorcluster)  [unwired: 11 in]
                      n285 = call "TrapBlankChan.vi"("error in (no error)"=w564) -> ("message"=w562:string, "error out"=w563:errorcluster)  [unwired: 9 in]
                    }
                    frame "Freq Out" {
                      n286 = call-poly <vilib>:"ULx Create Virtual Channel.vi"("frequency"="frequency", "duty cycle"="duty cycle", "counters"="ULx") -> ("task out"=w585:refnum<k24>, "error out"=w582:errorcluster)  [unwired: 11 in]
                      n287 = call "TrapBlankChan.vi"("error in (no error)"=w582) -> ("error out"=w581:errorcluster)  [unwired: 9 in, 1 out]
                      n288 = call-poly <vilib>:"ULx Create Virtual Channel.vi"("task in"=w585, "frequency"="frequency 2", "duty cycle"="duty cycle 2", "counters"="counters 13", "error in"=w581) -> ("task out"=w584:refnum<k24>, "error out"=w580:errorcluster)  [unwired: 9 in]
                      n289 = call "TrapBlankChan.vi"("error in (no error)"=w580) -> ("error out"=w579:errorcluster)  [unwired: 9 in, 1 out]
                      n290 = call-poly <vilib>:"ULx Create Virtual Channel.vi"("task in"=w584, "frequency"="frequency 3", "duty cycle"="duty cycle 3", "counters"="counters 14", "error in"=w579) -> ("task out"=w583:refnum<k24>, "error out"=w578:errorcluster)  [unwired: 9 in]
                      n291 = call "TrapBlankChan.vi"("error in (no error)"=w578) -> ("message"=w576:string, "error out"=w577:errorcluster)  [unwired: 9 in]
                    }
                    frame "Time Out" {
                      n292 = call-poly <vilib>:"ULx Create Virtual Channel.vi"("high time"="high time", "low time"="low time", "counters"="ULx") -> ("task out"=w604:refnum<k24>, "error out"=w602:errorcluster)  [unwired: 11 in]
                      n293 = call "TrapBlankChan.vi"("error in (no error)"=w602) -> ("error out"=w601:errorcluster)  [unwired: 9 in, 1 out]
                      n294 = call-poly <vilib>:"ULx Create Virtual Channel.vi"("task in"=w604, "high time"="high time 2", "low time"="low time 2", "counters"="counters 18", "error in"=w601) -> ("task out"=w603:refnum<k24>, "error out"=w600:errorcluster)  [unwired: 9 in]
                      n295 = call "TrapBlankChan.vi"("error in (no error)"=w600) -> ("error out"=w599:errorcluster)  [unwired: 9 in, 1 out]
                      n296 = call-poly <vilib>:"ULx Create Virtual Channel.vi"("task in"=w603, "high time"="high time 3", "low time"="low time 3", "counters"="counters 19", "error in"=w599) -> ("task out"=w597:refnum<k24>, "error out"=w598:errorcluster)  [unwired: 9 in]
                      n297 = call "TrapBlankChan.vi"("error in (no error)"=w598) -> ("message"=w595:string, "error out"=w596:errorcluster)  [unwired: 9 in]
                    }
                    frame "Ticks Out" {
                      n298 = call-poly <vilib>:"ULx Create Virtual Channel.vi"("high ticks"="high ticks", "low ticks"="low ticks", "counters"="ULx") -> ("task out"=w623:refnum<k24>, "error out"=w621:errorcluster)  [unwired: 11 in]
                      n299 = call "TrapBlankChan.vi"("error in (no error)"=w621) -> ("error out"=w620:errorcluster)  [unwired: 9 in, 1 out]
                      n300 = call-poly <vilib>:"ULx Create Virtual Channel.vi"("task in"=w623, "high ticks"="high ticks 2", "low ticks"="low ticks 2", "counters"="counters 16", "error in"=w620) -> ("task out"=w622:refnum<k24>, "error out"=w619:errorcluster)  [unwired: 9 in]
                      n301 = call "TrapBlankChan.vi"("error in (no error)"=w619) -> ("error out"=w618:errorcluster)  [unwired: 9 in, 1 out]
                      n302 = call-poly <vilib>:"ULx Create Virtual Channel.vi"("task in"=w622, "high ticks"="high ticks 3", "low ticks"="low ticks 3", "counters"="counters 20", "error in"=w618) -> ("task out"=w616:refnum<k24>, "error out"=w617:errorcluster)  [unwired: 9 in]
                      n303 = call "TrapBlankChan.vi"("error in (no error)"=w617) -> ("message"=w614:string, "error out"=w615:errorcluster)  [unwired: 9 in]
                    }
                  }
                }
                frame "DAQmx" {
                  n304 = case shown="\"Freq In\", Default" "xCntrType" {
                    tunnel: [w667 w702 w722 w753 w778 w787 w818] -> w628
                    tunnel: [w668 w703 w726 w754 w779 w788 w819] -> w627
                    tunnel: [w655 w709 w725 w742 w775 w789 w820] -> w626
                    frame "Freq In", Default {
                      n305 = call "FreqMM.vi"("measurement method"="measurement method") -> ("meastime vis"=w630:bool, "divisor vis"=w631:bool)
                      n306 = property on="measurement time" class="DigNum (strict)"("Visible"=w630) -> ()  [unwired: 2 in, 2 out]
                      n307 = call-poly <vilib>:"DAQmx Create Virtual Channel.vi"("maximum value"="max", "minimum value"="min", "measurement method"="measurement method", "counter"="DAQmx", "divisor"="divisor", "units"="units", "starting edge"="start edge", "measurement time"="measurement time") -> ("task out"=w657:refnum<k21>, "error out"=w669:errorcluster)  [unwired: 6 in]
                      n308 = property on="divisor" class="DigNum (strict)"("Visible"=w631) -> ()  [unwired: 2 in, 2 out]
                      n309 = call "NITrapBlankChan.vi"("error in (no error)"=w669) -> ("error out"=w659:errorcluster)  [unwired: 9 in, 1 out]
                      n310 = call-poly <vilib>:"DAQmx Create Virtual Channel.vi"("task in"=w657, "maximum value"="max", "minimum value"="min 21", "measurement method"="measurement method", "counter"="DAQmx", "divisor"="divisor 5", "units"="units", "error in"=w659, "starting edge"="start edge", "measurement time"="measurement time 2") -> ("task out"=w653:refnum<k21>, "error out"=w654:errorcluster)  [unwired: 4 in]
                      n311 = call "FreqMM.vi"("measurement method"="measurement method") -> ("meastime vis"=w642:bool, "divisor vis"=w641:bool)
                      n312 = call "NITrapBlankChan.vi"("error in (no error)"=w654) -> ("error out"=w658:errorcluster)  [unwired: 9 in, 1 out]
                      n313 = property on="measurement time 2" class="DigNum (strict)"("Visible"=w642) -> ()  [unwired: 2 in, 2 out]
                      n314 = call "FreqMM.vi"("measurement method"="measurement method") -> ("meastime vis"=w632:bool, "divisor vis"=w633:bool)
                      n315 = call-poly <vilib>:"DAQmx Create Virtual Channel.vi"("task in"=w653, "maximum value"="max", "minimum value"="min 24", "measurement method"="measurement method", "counter"="DAQmx", "divisor"="divisor 6", "units"="units", "error in"=w658, "starting edge"="start edge", "measurement time"="measurement time 3") -> ("task out"=w655:refnum<k21>, "error out"=w656:errorcluster)  [unwired: 4 in]
                      n316 = property on="divisor 5" class="DigNum (strict)"("Visible"=w641) -> ()  [unwired: 2 in, 2 out]
                      n317 = call "NITrapBlankChan.vi"("error in (no error)"=w656) -> ("message"=w667:string, "error out"=w668:errorcluster)  [unwired: 9 in]
                      n318 = property on="measurement time 3" class="DigNum (strict)"("Visible"=w632) -> ()  [unwired: 2 in, 2 out]
                      n319 = property on="divisor 6" class="DigNum (strict)"("Visible"=w633) -> ()  [unwired: 2 in, 2 out]
                    }
                    frame "Period In" {
                      n320 = call "FreqMM.vi"("measurement method"="measurement method") -> ("meastime vis"=w692:bool, "divisor vis"=w689:bool)
                      n321 = property on="measure time 6" class="DigNum (strict)"("Visible"=w692) -> ()  [unwired: 2 in, 2 out]
                      n322 = property on="divisor" class="DigNum (strict)"("Visible"=w689) -> ()  [unwired: 2 in, 2 out]
                      n323 = call-poly <vilib>:"DAQmx Create Virtual Channel.vi"("maximum value"="max", "minimum value"="min", "measurement method"="measurement method", "counter"="DAQmx", "divisor"="divisor", "units"="units", "starting edge"="start edge", "measurement time"="measure time 6") -> ("task out"=w699:refnum<k21>, "error out"=w698:errorcluster)  [unwired: 6 in]
                      n324 = call "NITrapBlankChan.vi"("error in (no error)"=w698) -> ("error out"=w707:errorcluster)  [unwired: 9 in, 1 out]
                      n325 = call "FreqMM.vi"("measurement method"="measurement method") -> ("meastime vis"=w681:bool, "divisor vis"=w679:bool)
                      n326 = call-poly <vilib>:"DAQmx Create Virtual Channel.vi"("task in"=w699, "maximum value"="max", "minimum value"="min", "measurement method"="measurement method", "counter"="DAQmx", "divisor"="divisor 2", "units"="units", "error in"=w707, "starting edge"="start edge", "measurement time"="measure time 7") -> ("task out"=w708:refnum<k21>, "error out"=w706:errorcluster)  [unwired: 4 in]
                      n327 = call "NITrapBlankChan.vi"("error in (no error)"=w706) -> ("error out"=w705:errorcluster)  [unwired: 9 in, 1 out]
                      n328 = property on="measure time 7" class="DigNum (strict)"("Visible"=w681) -> ()  [unwired: 2 in, 2 out]
                      n329 = call "FreqMM.vi"("measurement method"="measurement method") -> ("meastime vis"=w672:bool, "divisor vis"=w670:bool)
                      n330 = call-poly <vilib>:"DAQmx Create Virtual Channel.vi"("task in"=w708, "maximum value"="max", "minimum value"="min", "measurement method"="measurement method", "counter"="DAQmx", "divisor"="divisor 3", "units"="units", "error in"=w705, "starting edge"="start edge", "measurement time"="measure time 8") -> ("task out"=w709:refnum<k21>, "error out"=w704:errorcluster)  [unwired: 4 in]
                      n331 = property on="divisor 2" class="DigNum (strict)"("Visible"=w679) -> ()  [unwired: 2 in, 2 out]
                      n332 = call "NITrapBlankChan.vi"("error in (no error)"=w704) -> ("message"=w702:string, "error out"=w703:errorcluster)  [unwired: 9 in]
                      n333 = property on="divisor 3" class="DigNum (strict)"("Visible"=w670) -> ()  [unwired: 2 in, 2 out]
                      n334 = property on="measure time 8" class="DigNum (strict)"("Visible"=w672) -> ()  [unwired: 2 in, 2 out]
                    }
                    frame "Edge In" {
                      n335 = call-poly <vilib>:"DAQmx Create Virtual Channel.vi"("initial count"="init count", "count direction"="direction", "edge"="edge", "counter"="DAQmx") -> ("task out"=w724:refnum<k21>, "error out"=w731:errorcluster)  [unwired: 10 in]
                      n336 = call "NITrapBlankChan.vi"("error in (no error)"=w731) -> ("error out"=w730:errorcluster)  [unwired: 9 in, 1 out]
                      n337 = call-poly <vilib>:"DAQmx Create Virtual Channel.vi"("task in"=w724, "initial count"="init count 2", "count direction"="direction 7", "edge"="edge 7", "counter"="counter 8", "error in"=w730) -> ("task out"=w723:refnum<k21>, "error out"=w729:errorcluster)  [unwired: 8 in]
                      n338 = call "NITrapBlankChan.vi"("error in (no error)"=w729) -> ("error out"=w728:errorcluster)  [unwired: 9 in, 1 out]
                      n339 = call-poly <vilib>:"DAQmx Create Virtual Channel.vi"("task in"=w723, "initial count"="init count 3", "count direction"="direction 8", "edge"="edge 8", "counter"="counter 9", "error in"=w728) -> ("task out"=w725:refnum<k21>, "error out"=w727:errorcluster)  [unwired: 8 in]
                      n340 = call "NITrapBlankChan.vi"("error in (no error)"=w727) -> ("message"=w722:string, "error out"=w726:errorcluster)  [unwired: 9 in]
                    }
                    frame "Position In" {
                      n341 = call-poly <vilib>:"DAQmx Create Virtual Channel.vi"("z index enable"="z index", "z index value"="z value", "z index phase"="z phase", "counter"="DAQmx", "decoding type"="type", "units"="units", "pulses per revolution"="pulses per revolution", "initial angle"="initial angle\npulses per") -> ("task out"=w750:refnum<k21>, "error out"=w752:errorcluster)  [unwired: 6 in]
                      n342 = call "NITrapBlankChan.vi"("error in (no error)"=w752) -> ("error out"=w751:errorcluster)  [unwired: 9 in, 1 out]
                      n343 = call-poly <vilib>:"DAQmx Create Virtual Channel.vi"("task in"=w750, "z index enable"="z index  2", "z index value"="z value 2", "z index phase"="z phase 2", "counter"="counter 11", "decoding type"="type", "units"="units 22", "error in"=w751, "pulses per revolution"="pulses per revolution 2", "initial angle"="initial angle\npulses per") -> ("task out"=w742:refnum<k21>, "error out"=w741:errorcluster)  [unwired: 4 in]
                      n344 = call "NITrapBlankChan.vi"("error in (no error)"=w741) -> ("message"=w753:string, "error out"=w754:errorcluster)  [unwired: 9 in]
                    }
                    frame "Freq Out" {
                      n345 = call-poly <vilib>:"DAQmx Create Virtual Channel.vi"("frequency"="frequency", "duty cycle"="duty cycle", "counter"="DAQmx", "idle state"="idle state", "initial delay"="initial delay") -> ("task out"=w776:refnum<k21>, "error out"=w777:errorcluster)  [unwired: 9 in]
                      n346 = call "NITrapBlankChan.vi"("error in (no error)"=w777) -> ("error out"=w773:errorcluster)  [unwired: 9 in, 1 out]
                      n347 = call-poly <vilib>:"DAQmx Create Virtual Channel.vi"("task in"=w776, "frequency"="frequency 5", "duty cycle"="duty cycle 5", "counter"="counter 13", "error in"=w773, "idle state"="idle state 5", "initial delay"="initial delay 5") -> ("task out"=w774:refnum<k21>, "error out"=w772:errorcluster)  [unwired: 7 in]
                      n348 = call "NITrapBlankChan.vi"("error in (no error)"=w772) -> ("error out"=w771:errorcluster)  [unwired: 9 in, 1 out]
                      n349 = call-poly <vilib>:"DAQmx Create Virtual Channel.vi"("task in"=w774, "frequency"="frequency 6", "duty cycle"="duty cycle 6", "counter"="counter 14", "error in"=w771, "idle state"="idle state 4", "initial delay"="initial delay 4") -> ("task out"=w775:refnum<k21>, "error out"=w770:errorcluster)  [unwired: 7 in]
                      n350 = call "NITrapBlankChan.vi"("error in (no error)"=w770) -> ("message"=w778:string, "error out"=w779:errorcluster)  [unwired: 9 in]
                    }
                    frame "Time Out" {
                      n351 = call-poly <vilib>:"DAQmx Create Virtual Channel.vi"("high time"="high time", "low time"="low time", "counter"="DAQmx", "idle state"="idle state", "initial delay"="initial delay") -> ("task out"=w803:refnum<k21>, "error out"=w804:errorcluster)  [unwired: 9 in]
                      n352 = call "NITrapBlankChan.vi"("error in (no error)"=w804) -> ("error out"=w801:errorcluster)  [unwired: 9 in, 1 out]
                      n353 = call-poly <vilib>:"DAQmx Create Virtual Channel.vi"("task in"=w803, "high time"="high time 5", "low time"="low time 5", "counter"="counter 16", "error in"=w801, "idle state"="idle state 9", "initial delay"="initial delay 8") -> ("task out"=w802:refnum<k21>, "error out"=w800:errorcluster)  [unwired: 7 in]
                      n354 = call "NITrapBlankChan.vi"("error in (no error)"=w800) -> ("error out"=w799:errorcluster)  [unwired: 9 in, 1 out]
                      n355 = call-poly <vilib>:"DAQmx Create Virtual Channel.vi"("task in"=w802, "high time"="high time 6", "low time"="low time 6", "counter"="counter 17", "error in"=w799, "idle state"="idle state 8", "initial delay"="initial delay 7") -> ("task out"=w789:refnum<k21>, "error out"=w798:errorcluster)  [unwired: 7 in]
                      n356 = call "NITrapBlankChan.vi"("error in (no error)"=w798) -> ("message"=w787:string, "error out"=w788:errorcluster)  [unwired: 9 in]
                    }
                    frame "Ticks Out" {
                      n357 = call-poly <vilib>:"DAQmx Create Virtual Channel.vi"("high ticks"="high ticks", "low ticks"="low ticks", "counter"="DAQmx", "source of ticks"="source of ticks", "idle state"="idle state", "initial delay"="initial delay") -> ("task out"=w831:refnum<k21>, "error out"=w832:errorcluster)  [unwired: 8 in]
